vi "Distribute.vi"(8 "error in (no error)":errorcluster, 10 "Bounds":T1, 11 "Container in":refnum<class "Divider.lvclass">) -> (0 "error out":errorcluster, 2 "Bounds":T1[](array[typedef]), 3 "Container out":refnum<class "Divider.lvclass">, 5 "Visible bounds":T1[](array[typedef]), 7 "Visible indices":i32[](array[numeric]))   [LabVIEW 2013, in "Divider.lvclass"]
doc: "Copyright 2018, Wiebe Walstra, wiebe@carya.nl."
uses:
  Divider.lvclass
  <vilib>/Utility/miscctls.llb/LVRectTypeDef.ctl
  Divider.lvclass/Divider.ctl
  IContainer.lvclass
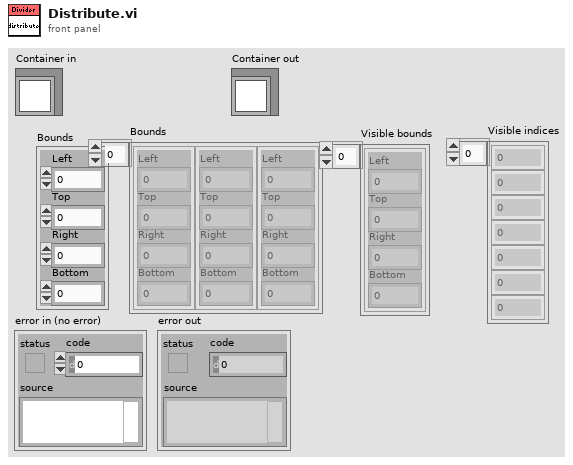
[diagram p1: front panel]
types:
  T1 = typedef "LVRectTypeDef.ctl" = cluster{"Left":i16, "Top":i16, "Right":i16, "Bottom":i16}
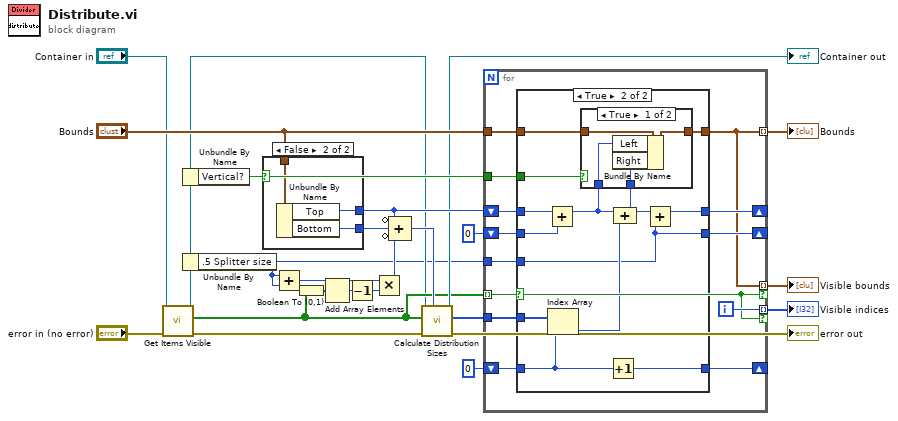
[diagram p0: block diagram]
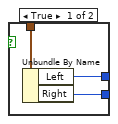
[diagram p2: hidden frame]
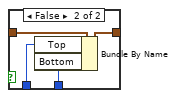
[diagram p4: hidden frame]
diagram:
  n1 = call "Get Items Visible.vi"("error in (no error)"="error in (no error)", "IContainer in"="Container in") -> ("error out"=w4:errorcluster, "Visible"=w5:bool[], "IContainer out"=w3:refnum<class "Divider.lvclass">)  [unwired: 6 in, 1 out]
  n2 = Unbundle By Name(w3) -> ("Vertical?"=w20:bool)
  n3 = Unbundle By Name(w3) -> (".5 Splitter size"=w1:i16)
  n4 = case shown="False" w20 {
    tunnel: [w27 w30] -> w23
    tunnel: "Bounds" -> [w26 w29]
    tunnel: [w25 w28] -> w13
    frame True {
      n5 = Unbundle By Name(w26) -> ("Left"=w27:i16, "Right"=w25:i16)
    }
    frame False {
      n6 = Unbundle By Name(w29) -> ("Top"=w30:i16, "Bottom"=w28:i16)
    }
  }
  n7 = Add(x=w1, y=w1) -> (x+y=w2:i16)
  n8 = Boolean To (0,1)(Boolean=w5) -> (0, 1=w12:i16[])
  n9 = Add Array Elements(numeric array=w12) -> (sum=w11:i16)
  n10 = Decrement(x=w11) -> (x-1=w10:i16)
  n11 = Multiply(x=w2, y=w10) -> (x*y=w8:i16)
  n12 = Compound Arithmetic op=ADD(invert w23, w13, invert w8) -> (w18:i16)
  n13 = call "Calculate Distribution Sizes.vi"("size"=w18, "error in (no error)"=w4, "Visible"=w5, "Container in"=w3) -> ("error out"=→"error out":errorcluster, "Start"=w9:i16[], "Container out"=→"Container out":refnum<class "Divider.lvclass">)  [unwired: 5 in]
  n14 = for {
    shift-right: [w41] -> _
    shift-left: w23 -> [w42]
    tunnel: "Bounds" -> [w43]
    tunnel: [w33] -> w21 mode=indexing
    tunnel: w20 -> [w40]
    tunnel: w5 -> [w32] mode=indexing
    tunnel: w9 -> [w39]
    shift-right: [w37] -> _
    shift-left: 0 -> [w38]
    tunnel: [w33] -> w14 mode=indexing if=w32
    shift-right: [w35] -> _
    shift-left: i16 0 -> [w36]
    tunnel: [w34] -> w6 mode=indexing if=w32
    tunnel: w1 -> [w31]
    i -> [w34]
    n15 = case shown="True" w32 {
      tunnel: w43 -> [w46 w60]
      tunnel: w42 -> [w47 w52]
      tunnel: [w47 w51] -> w41
      tunnel: [w46 w58] -> w33
      tunnel: w40 -> [_ w57]
      tunnel: w39 -> [_ w56]
      tunnel: w38 -> [w45 w55]
      tunnel: [w45 w54] -> w37
      tunnel: w36 -> [w44 w49]
      tunnel: [w44 w48] -> w35
      tunnel: w31 -> [_ w48]
      frame False {
      }
      frame True {
        n16 = Add(x=w52, y=w49) -> (x+y=w50:i16)
        n17 = Index Array(array=w56, index=w55) -> (element=w53:i16)
        n18 = Increment(x=w55) -> (x+1=w54:i32)
        n19 = Compound Arithmetic op=ADD(w50, w53) -> (w59:i16)
        n20 = case shown="True" w57 {
          tunnel: w60 -> [w64 w68]
          tunnel: w50 -> [w63 w67]
          tunnel: w59 -> [w62 w66]
          tunnel: [w61 w65] -> w58
          frame True {
            n21 = Bundle By Name(cluster=w64, "Left"=w63, "Right"=w62) -> (w61:T1)
          }
          frame False {
            n22 = Bundle By Name(cluster=w68, "Top"=w67, "Bottom"=w66) -> (w65:T1)
          }
        }
        n23 = Add(x=w59, y=w48) -> (x+y=w51:i16)
      }
    }
  }
  "Bounds" <- w21
  "Visible bounds" <- w14
  "Visible indices" <- w6
